vi "Get Request example.vi"() -> ()   [LabVIEW 2016]
panel:
  out "data":T1(array[cluster])
  in  "Team":T2(ring)=enum."Researchers"
  in  "error in (no error)":errorcluster
  out "error out":errorcluster
  in  "Authentication Info":T3={"Client ID"="", "Client Secret"="", "Redirect URI"="", "Token Endpoint"="https://app.asana.com/-/oauth_token", "Scope"=""}
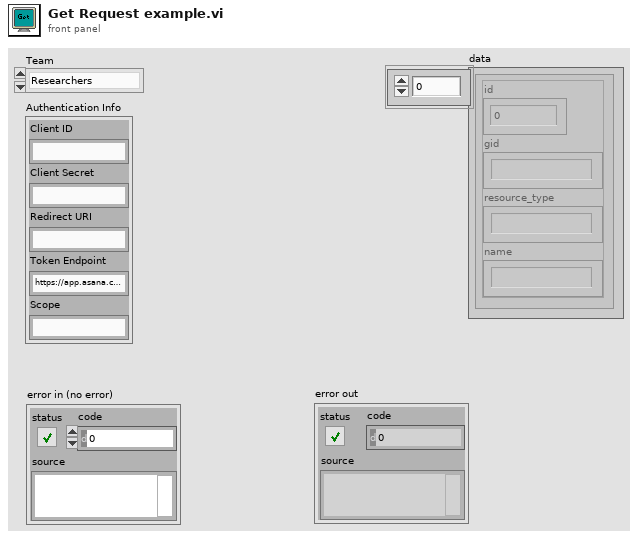
[diagram p1: front panel]
types:
  T1 = cluster{"id":i64, "gid":string, "resource_type":string, "name":string}[]
  T2 = enum16{"GSR", "Research Projects", "Undergrads", "Researchers", "Hardware", "Software", "LevyLab", "Samples", "Manuscripts", "AoT", "WorkStudy"}
  T3 = cluster{"Client ID":string, "Client Secret":string, "Redirect URI":string, "Token Endpoint":string, "Scope":string}
  T4 = typedef "REST Client.lvlib/REST Client.lvclass/HTTP Header.ctl" = cluster{"header":string, "value":string}
  T5 = cluster{"gid":string, "name":string, "resource_type":string}[]
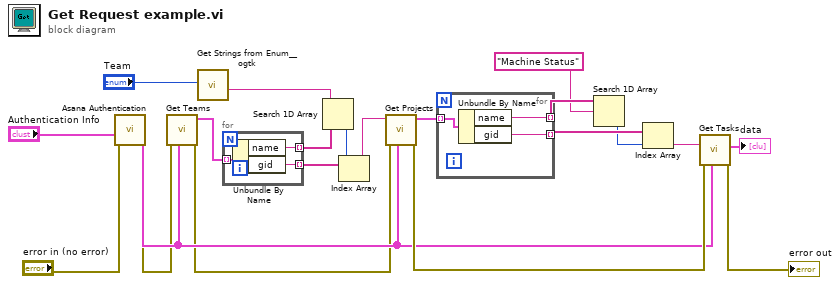
[diagram p0: block diagram]
diagram:
  n1 = call "Asana Authentication.vi"("error in (no error)"="error in (no error)", "Authentication Info"="Authentication Info") -> ("error out"=w9:errorcluster, "Authentication Header"=w12:T4[])  [unwired: 6 in, 2 out]
  n2 = call "Get Teams.vi"("Authorization"=w12, "error in (no error)"=w9) -> ("error out"=w10:errorcluster, "Teams Out"=w6:T5)  [unwired: 8 in]
  n3 = call <userlib>:"Get Strings from Enum__ogtk.vi"("Enum"="Team") -> ("String Value"=w7:string)  [unwired: 7 in, 3 out]
  n4 = for {
    tunnel: w6 -> [w24] mode=indexing
    tunnel: [w23] -> w5 mode=indexing
    tunnel: [w22] -> w4 mode=indexing
    n5 = Unbundle By Name(w24) -> ("name"=w23:string, "gid"=w22:string)
  }
  n6 = Search 1D Array(1D array=w5, element=w7) -> (index of element=w3:i32)  [unwired: 1 in]
  n7 = Index Array(array=w4, index=w3) -> (element=w2:string)
  n8 = call "Get Projects.vi"("Authorization"=w12, "error in (no error)"=w10, "Team GID"=w2) -> ("error out"=w15:errorcluster, "Projects Out"=w13:T5)  [unwired: 7 in]
  n9 = for {
    tunnel: w13 -> [w27] mode=indexing
    tunnel: [w26] -> w18 mode=indexing
    tunnel: [w25] -> w20 mode=indexing
    n10 = Unbundle By Name(w27) -> ("name"=w26:string, "gid"=w25:string)
  }
  n11 = Search 1D Array(1D array=w18, element="Machine Status") -> (index of element=w19:i32)  [unwired: 1 in]
  n12 = Index Array(array=w20, index=w19) -> (element=w16:string)
  n13 = call "Get Tasks.vi"("Authorization"=w12, "error in (no error)"=w15, "Project GID"=w16) -> ("error out"=→"error out":errorcluster, "data"=→"data":T1)  [unwired: 7 in]
